vi "Init_ctl_refs.vi"(11 "VI Refnum":refnum<vi>) -> ()   [LabVIEW 2019]
uses:
  Typedefs/Cluster_refs_controles.ctl
panel:
  out "Ctl Refnum":refnum<vi>
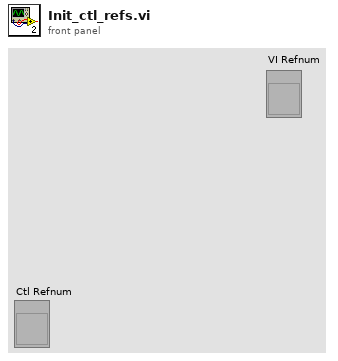
[diagram p1: front panel]
types:
  T1 = typedef "Cluster_refs_controles.ctl" = cluster{"Comenzar mov":refnum<vi>, "Home":refnum<vi>, "Izq":refnum<vi>, "Der":refnum<vi>, "Stop Program":refnum<vi>, "Avanzar":refnum<vi>, "Bajar Z":refnum<vi>, "Distancia":refnum<vi>, "Subir Z":refnum<vi>, "Retroc":refnum<vi>, "Estado arduino":refnum<vi>}
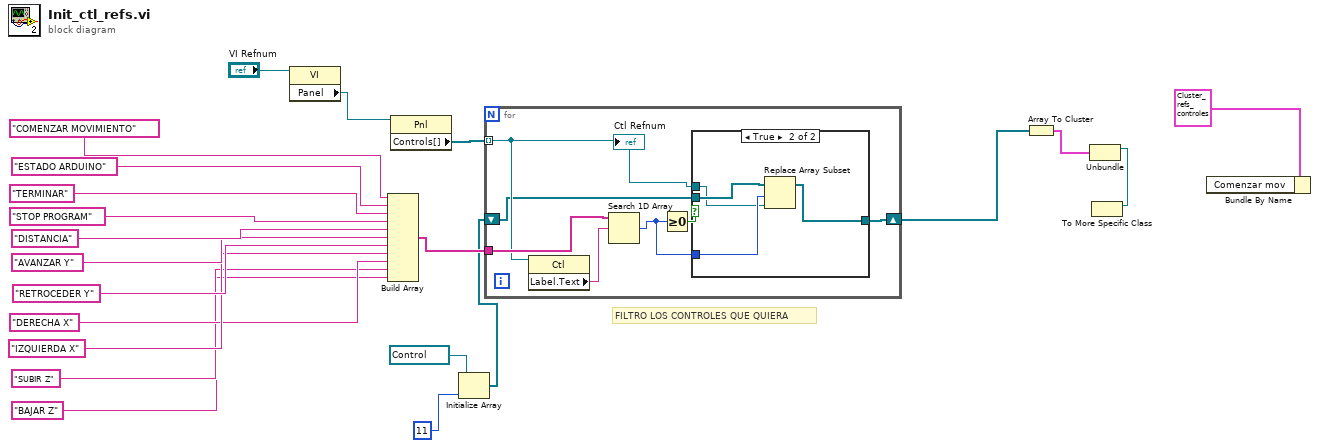
[diagram p0: block diagram]
diagram:
  # "FILTRO LOS CONTROLES QUE QUIERA"
  n1 = property class="VI"(reference="VI Refnum") -> ("Panel"=w22:refnum<vi>)  [unwired: 1 in, 2 out]
  n2 = Build Array("COMENZAR MOVIMIENTO", "ESTADO ARDUINO" ("element"), "TERMINAR" ("element"), "STOP PROGRAM" ("element"), "DISTANCIA" ("element"), "AVANZAR Y" ("element"), "RETROCEDER Y" ("element"), "IZQUIERDA X" ("element"), "DERECHA X" ("element"), "SUBIR Z" ("element"), "BAJAR Z" ("element")) -> (w18:string[])
  n3 = property class="Pnl"(reference=w22) -> ("Controls[]"=w21:refnum<vi>[])  [unwired: 1 in, 2 out]
  n4 = Initialize Array(refnum<vi> refnum ("Ctl Refnum"), 11 ("dimension size")) -> (w15:refnum<vi>[])
  n5 = for {
    tunnel: w21 -> [w26] mode=indexing
    tunnel: w18 -> [w29]
    shift-right: [w24] -> w14
    shift-left: w15 -> [w25]
    n6 = property class="Ctl"(reference=w26) -> ("Label.Text"=w27:string)  [unwired: 1 in, 2 out]
    n7 = Search 1D Array(1D array=w29, element=w27) -> (index of element=w23:i32)  [unwired: 1 in]
    n8 = Greater Or Equal To 0?(x=w23) -> (x >= 0?=w28:bool)
    n9 = case shown="True" w28 {
      tunnel: w26 -> [_ w31]
      tunnel: w25 -> [w30 w34]
      tunnel: [w30 w33] -> w24
      tunnel: w23 -> [_ w32]
      frame False {
      }
      frame True {
        n10 = Replace Array Subset(array=w34, new element=w31, index=w32) -> (w33:refnum<vi>[])
      }
    }
    "Ctl Refnum" <- w26
  }
  n11 = Array To Cluster(array=w14) -> (cluster=w3:cluster{"[0]":refnum<vi>, "[1]":refnum<vi>})
  n12 = Unbundle(w3) -> ("[0]"=w2:refnum<vi>)  [unwired: 1 out]
  n13 = To More Specific Class(reference=w2) -> ()  [unwired: 2 in, 2 out]
  n14 = Bundle By Name(cluster=T1 {"Comenzar mov"=refnum, "Home"=refnum, "Izq"=refnum, "Der"=refnum, "Stop Program"=refnum, "Avanzar"=refnum, "Bajar Z"=refnum, "Distancia"=refnum, "Subir Z"=refnum, "Retroc"=refnum, "Estado arduino"=refnum} ("Cluster de refs controles")) -> ()  [unwired: 1 in, 1 out]
